vi "Get Becker-Hickl Data Block Type.vi"(11 "Block Type":u16 format="%.0b") -> (0 "Compressed":bool, 3 "Data Block Type":T1)   [LabVIEW 2021, in "Becker-Hickl Files.lvlib"]
uses:
  Becker-Hickl Files.lvlib
  Becker-Hickl Data Block Type.ctl
  Becker-Hickl Data Creation Mode.ctl
  Becker-Hickl Data Block Content.ctl
  Becker-Hickl Data Type.ctl
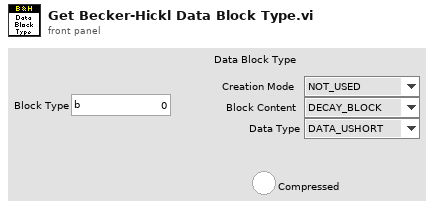
[diagram p1: front panel]
types:
  T1 = typedef "Becker-Hickl Files.lvlib/Becker-Hickl Data Block Type.ctl" = cluster{"Creation Mode":T2, "Block Content":T3, "Data Type":T4}
  T2 = typedef "Becker-Hickl Files.lvlib/Becker-Hickl Data Creation Mode.ctl" = enum16{"NOT_USED", "MEAS_DATA", "FLOW_DATA", "MEAS_DATA_FROM_FILE", "CALC_DATA", "SIM_DATA", "FIFO_DATA", "FIFO_DATA_FROM_FILE"}
  T3 = typedef "Becker-Hickl Files.lvlib/Becker-Hickl Data Block Content.ctl" = enum16{"DECAY_BLOCK", "PAGE_BLOCK", "FCS_BLOCK", "FIDA_BLOCK", "FILDA_BLOCK", "MCS_BLOCK", "IMG_BLOCK"}
  T4 = typedef "Becker-Hickl Files.lvlib/Becker-Hickl Data Type.ctl" = enum16{"DATA_USHORT", "DATA_ULONG", "DATA_DBL"}
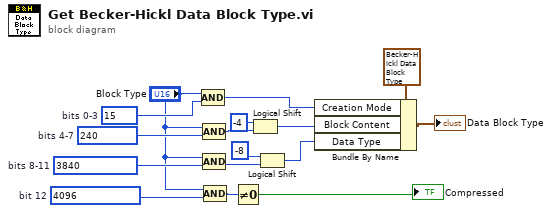
[diagram p0: block diagram]
diagram:
  w4 = u16 4096  # bit 12
  w12 = u16 3840  # bits 8-11
  w15 = u16 240  # bits 4-7
  w16 = u16 15  # bits 0-3
  n1 = Compound Arithmetic op=AND("Block Type", w16) -> (w8:u16)
  n2 = Compound Arithmetic op=AND("Block Type", w15) -> (w14:u16)
  n3 = Compound Arithmetic op=AND("Block Type", w12) -> (w11:u16)
  n4 = Compound Arithmetic op=AND("Block Type", w4) -> (w2:u16)
  n5 = Not Equal To 0?(x=w2) -> (x != 0?=→"Compressed":bool)
  n6 = Logical Shift(y=i16 -4, x=w14) -> (x << y=w9:u16)
  n7 = Logical Shift(y=i16 -8, x=w11) -> (x << y=w7:u16)
  n8 = Bundle By Name(cluster=T1 {"Creation Mode"=enum."NOT_USED", "Block Content"=enum."DECAY_BLOCK", "Data Type"=enum."DATA_USHORT"} ("Data Block Type"), "Creation Mode"=w8, "Block Content"=w9, "Data Type"=w7) -> (→"Data Block Type":T1)
